vi "DAQMx Channels DAO.vi"(7 "Config Ref  In":T1, 8 "error in (no error)":errorcluster, 9 "Names In":T2, 11 "Actions":T3) -> (0 "error out":errorcluster, 1 "Names Out":T2, 4 "Config Ref Out":T1)   [LabVIEW 2013]
uses:
  Metadata/Persistant DAO Actions.ctl
  <vilib>/Utility/config.llb/Config Data RefNum.ctl
  <vilib>/Utility/config.llb/Read Key (String).vi
  <vilib>/Utility/config.llb/Write Key (String).vi
  <vilib>/Utility/config.llb/NI_LVConfig.lvlib
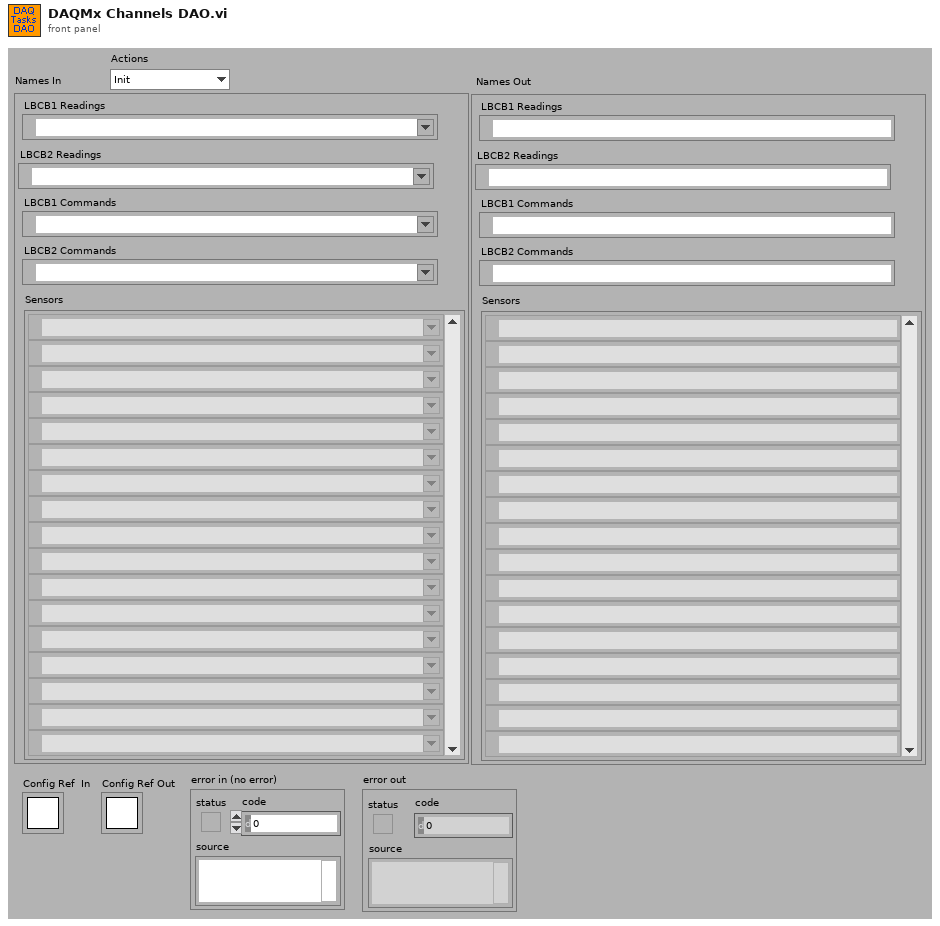
[diagram p1: front panel]
types:
  T1 = typedef "NI_LVConfig.lvlib/Config Data RefNum.ctl" = refnum<k1>
  T2 = cluster{"LBCB1 Readings":refnum<k21>, "LBCB2 Readings":refnum<k21>, "LBCB1 Commands":refnum<k21>, "LBCB2 Commands":refnum<k21>, "Sensors":refnum<k21>[]}
  T3 = typedef "Persistant DAO Actions.ctl" = enum16{"Init", "Get", "Set", "Load", "Save"}
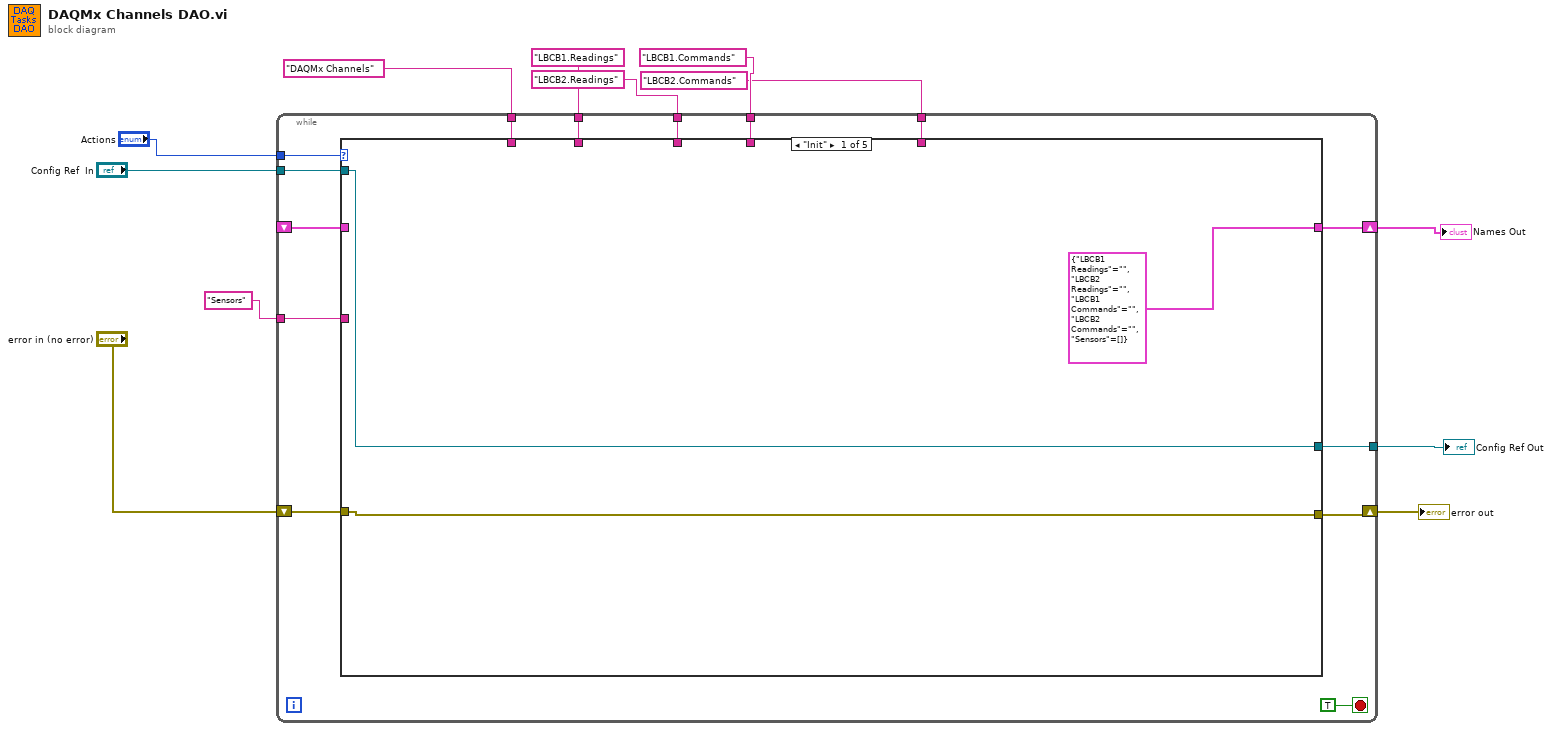
[diagram p0: block diagram]
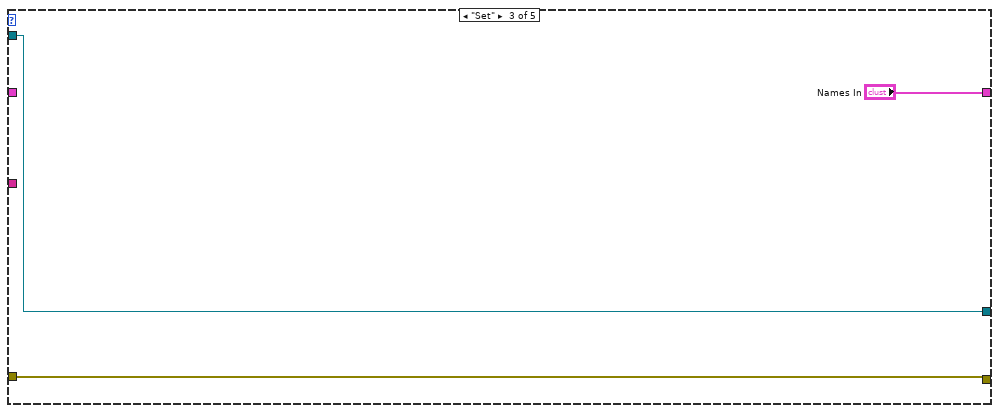
[diagram p3: hidden frame]
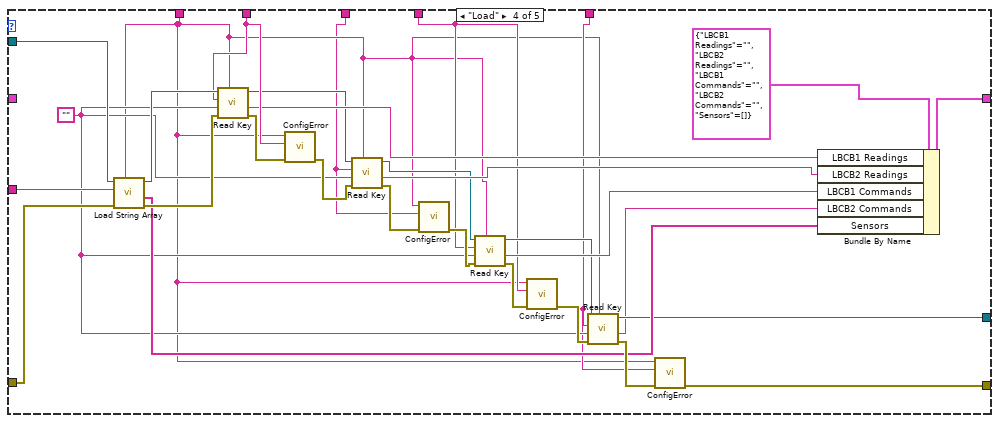
[diagram p4: hidden frame]
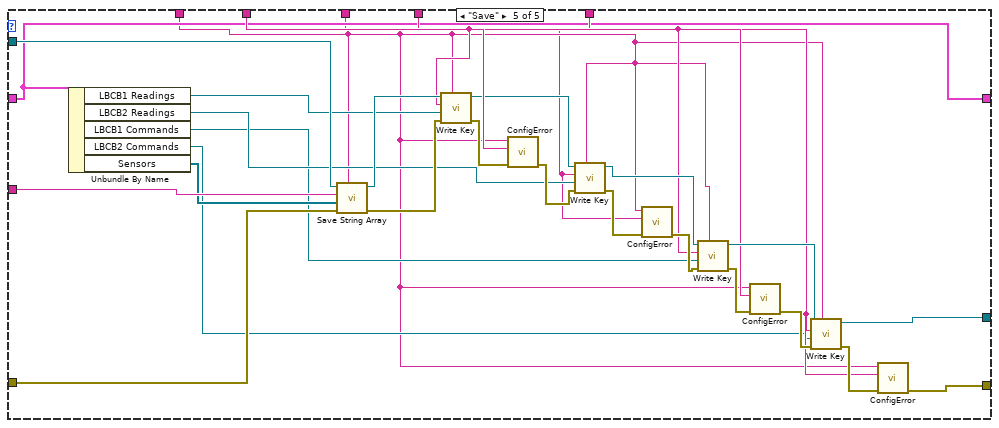
[diagram p5: hidden frame]
diagram:
  n1 = while {
    tunnel: "Actions" -> [w25]
    shift-right: [w24] -> w11
    shift-left: _ -> [w23]
    tunnel: "Config Ref  In" -> [w22]
    tunnel: "DAQMx Channels" ("section") -> [w21]
    shift-right: [w14] -> w1
    shift-left: "error in (no error)" -> [w20]
    tunnel: "Sensors" ("key") -> [w19]
    tunnel: "LBCB1.Readings" ("section") -> [w18]
    tunnel: "LBCB2.Readings" ("section") -> [w17]
    tunnel: "LBCB1.Commands" ("section") -> [w16]
    tunnel: "LBCB2.Commands" ("section") -> [w15]
    tunnel: [w13] -> w2
    stop <- TRUE stop-if-true
    n2 = case shown="\"Init\"" w25 {
      tunnel: [T2 {"LBCB1 Readings"="", "LBCB2 Readings"="", "LBCB1 Commands"="", "LBCB2 Commands"="", "Sensors"=[]} ("Names In") w32 "Names In" w57 w73] -> w24
      tunnel: w23 -> [_ w32 _ _ w73]
      tunnel: w22 -> [w27 w31 w34 w65 w93]
      tunnel: w21 -> [_ _ _ w37 w67]
      tunnel: w20 -> [w28 w30 w33 w64 w92]
      tunnel: w19 -> [_ _ _ w60 w88]
      tunnel: w18 -> [_ _ _ w59 w87]
      tunnel: w17 -> [_ _ _ w36 w66]
      tunnel: w16 -> [_ _ _ w39 w75]
      tunnel: w15 -> [_ _ _ w38 w74]
      tunnel: [w28 w30 w33 w42 w77] -> w14
      tunnel: [w27 w31 w34 w41 w76] -> w13
      frame "Init" {
      }
      frame "Get" {
      }
      frame "Set" {
      }
      frame "Load" {
        w45 = ""
        n3 = call "Load String Array.vi"("section"=w37, "error in (no error)"=w64, "key"=w60, "refnum"=w65) -> ("error out"=w62:errorcluster, "String Array Out"=w52:string[], "refnum out"=w61:T1)  [unwired: 5 out]
        n4 = call-poly <vilib>:"Read Key.vi"("section"=w37, "error in (no error)"=w62, "default value"=w45, "key"=w59, "refnum"=w61) -> ("error out"=w63:errorcluster, "value"=w56:string, "refnum out"=w50:T1)  [unwired: 1 in, 3 out]
        n5 = call "ConfigError.vi"("error in (no error)"=w63, "Key"=w59, "Section"=w37) -> ("error out"=w51:errorcluster)  [unwired: 8 out]
        n6 = call-poly <vilib>:"Read Key.vi"("section"=w37, "error in (no error)"=w51, "default value"=w45, "key"=w36, "refnum"=w50) -> ("error out"=w55:errorcluster, "value"=w49:string, "refnum out"=w43:T1)  [unwired: 1 in, 3 out]
        n7 = call "ConfigError.vi"("error in (no error)"=w55, "Key"=w36, "Section"=w37) -> ("error out"=w48:errorcluster)  [unwired: 8 out]
        n8 = call-poly <vilib>:"Read Key.vi"("section"=w37, "error in (no error)"=w48, "default value"=w45, "key"=w39, "refnum"=w43) -> ("error out"=w54:errorcluster, "value"=w47:string, "refnum out"=w44:T1)  [unwired: 1 in, 3 out]
        n9 = call "ConfigError.vi"("error in (no error)"=w54, "Key"=w39, "Section"=w37) -> ("error out"=w46:errorcluster)  [unwired: 8 out]
        n10 = call-poly <vilib>:"Read Key.vi"("section"=w37, "error in (no error)"=w46, "default value"=w45, "key"=w38, "refnum"=w44) -> ("error out"=w53:errorcluster, "value"=w40:string, "refnum out"=w41:T1)  [unwired: 1 in, 3 out]
        n11 = call "ConfigError.vi"("error in (no error)"=w53, "Key"=w38, "Section"=w37) -> ("error out"=w42:errorcluster)  [unwired: 8 out]
        n12 = Bundle By Name(cluster=T2 {"LBCB1 Readings"="", "LBCB2 Readings"="", "LBCB1 Commands"="", "LBCB2 Commands"="", "Sensors"=[]} ("Names In"), "LBCB1 Readings"=w56, "LBCB2 Readings"=w49, "LBCB1 Commands"=w47, "LBCB2 Commands"=w40, "Sensors"=w52) -> (w57:T2)
      }
      frame "Save" {
        n13 = Unbundle By Name(w73) -> ("LBCB1 Readings"=w72:refnum<k21>, "LBCB2 Readings"=w70:refnum<k21>, "LBCB1 Commands"=w69:refnum<k21>, "LBCB2 Commands"=w68:refnum<k21>, "Sensors"=w71:refnum<k21>[])
        n14 = call "Save String Array.vi"("section"=w67, "error in (no error)"=w92, "String Array In"=w71, "key"=w88, "refnum"=w93) -> ("error out"=w90:errorcluster, "refnum out"=w89:T1)  [unwired: 5 in]
        n15 = call-poly <vilib>:"Write Key.vi"("section"=w67, "error in (no error)"=w90, "value"=w72, "key"=w87, "refnum"=w89) -> ("error out"=w91:errorcluster, "refnum out"=w82:T1)  [unwired: 4 in, 1 out]
        n16 = call "ConfigError.vi"("error in (no error)"=w91, "Key"=w87, "Section"=w67) -> ("error out"=w83:errorcluster)  [unwired: 8 out]
        n17 = call-poly <vilib>:"Write Key.vi"("section"=w67, "error in (no error)"=w83, "value"=w70, "key"=w66, "refnum"=w82) -> ("error out"=w86:errorcluster, "refnum out"=w78:T1)  [unwired: 4 in, 1 out]
        n18 = call "ConfigError.vi"("error in (no error)"=w86, "Key"=w66, "Section"=w67) -> ("error out"=w81:errorcluster)  [unwired: 8 out]
        n19 = call-poly <vilib>:"Write Key.vi"("section"=w67, "error in (no error)"=w81, "value"=w69, "key"=w75, "refnum"=w78) -> ("error out"=w85:errorcluster, "refnum out"=w79:T1)  [unwired: 4 in, 1 out]
        n20 = call "ConfigError.vi"("error in (no error)"=w85, "Key"=w75, "Section"=w67) -> ("error out"=w80:errorcluster)  [unwired: 8 out]
        n21 = call-poly <vilib>:"Write Key.vi"("section"=w67, "error in (no error)"=w80, "value"=w68, "key"=w74, "refnum"=w79) -> ("error out"=w84:errorcluster, "refnum out"=w76:T1)  [unwired: 4 in, 1 out]
        n22 = call "ConfigError.vi"("error in (no error)"=w84, "Key"=w74, "Section"=w67) -> ("error out"=w77:errorcluster)  [unwired: 8 out]
      }
    }
  }
  "Names Out" <- w11
  "error out" <- w1
  "Config Ref Out" <- w2
